vi "niRFUtil LCAPI Copy 1D Array (1 WFM SGL).vi"(0 "Waveform In":T1[](array[typedef]) {"y" min=0 max=127 format="%.2f"; "dx" format="%^.2e"; "x0" format="%^.2e"}, 11 "error in (no error)":errorcluster, 12 "Data Copy Descriptor":u64) -> (4 "Waveform Out":T1[](array[typedef]) {"y" min=0 max=127 format="%.2f"; "dx" format="%^.2e"; "x0" format="%^.2e"}, 15 "error out":errorcluster)   [LabVIEW 2015, in "niRFUtil.lvlib"]
uses:
  niRFUtil.lvlib
  Includes/niRFUtil INC Real Waveform.ctl
  Includes/niRFUtil INC Real Array.ctl
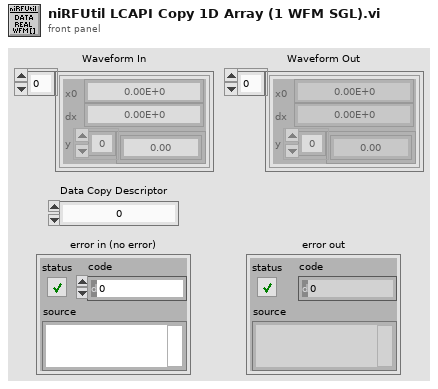
[diagram p1: front panel]
types:
  T1 = typedef "niRFUtil.lvlib/niRFUtil INC Real Waveform.ctl" = cluster{"x0":dbl, "dx":dbl, "y":T2}
  T2 = typedef "niRFUtil.lvlib/niRFUtil INC Real Array.ctl" = sgl[]
  T3 = cluster{"status":bool, "return type":i32, "errorString":string}
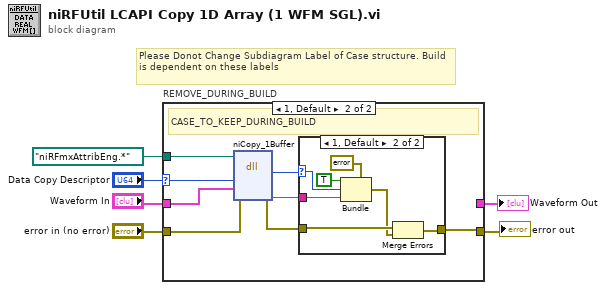
[diagram p0: block diagram]
diagram:
  # "Please Donot Change Subdiagram Label of Case structure. Build is dependent on these labels"
  n1 = case "REMOVE_DURING_BUILD" shown="1, Default" "Data Copy Descriptor" {
    selector: "Data Copy Descriptor" -> [_ w11]
    tunnel: "error in (no error)" -> [w7 w16]
    tunnel: "Waveform In" -> [w8 w15]
    tunnel: [w8 _] -> w3
    tunnel: [w7 w10] -> w2
    tunnel: path "niRFmxAttribEng.*" ("path in") -> [_ w9]
    frame 0 {
      # "Development"
    }
    frame 1, Default {
      # "CASE_TO_KEEP_DURING_BUILD"
      n2 = dll-call lib="niRFmxAttribEng.*" fn="niCopy_1Buffer"(path in=w9, error in=w16, "dataCopyDescriptor"=w11, "source"=w15) -> (error out=w12:errorcluster, "return type"=w13:i32, "errorString"=w14:string)  [unwired: 4 in, 1 out]
      n3 = case shown="1, Default" w13 {
        selector: w13 -> [_ w23]
        tunnel: w14 -> [_ w22]
        tunnel: w12 -> [w17 w20]
        tunnel: [w17 w21] -> w10
        frame 0 {
        }
        frame 1, Default {
          n4 = Bundle(cluster=T3 {"status"=FALSE, "return type"=0, "errorString"=""}, "status"=TRUE, "return type"=w23, "errorString"=w22) -> (w19:T3)
          n5 = Merge Errors(w20, w19) -> (w21:errorcluster)
        }
      }
    }
  }
  "Waveform Out" <- w3
  "error out" <- w2
